vi "BISS_ReadConfigFile.vi"() -> ()   [LabVIEW 2019]
uses:
  DUT_Interface/lv_interface/MHM_1SL_interface.lvlib
panel:
  out "pulEnSsi":u32
  in  "pcFilename":string="test.cfg"
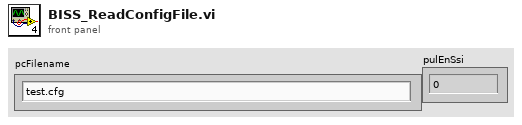
[diagram p1: front panel]
types:
  T1 = enum16{"MHM_NO_INTERFACE", "MHM_MB3U_SPI", "MHM_MB3U_BISS", "MHM_MB4U", "MHM_MB5U"}
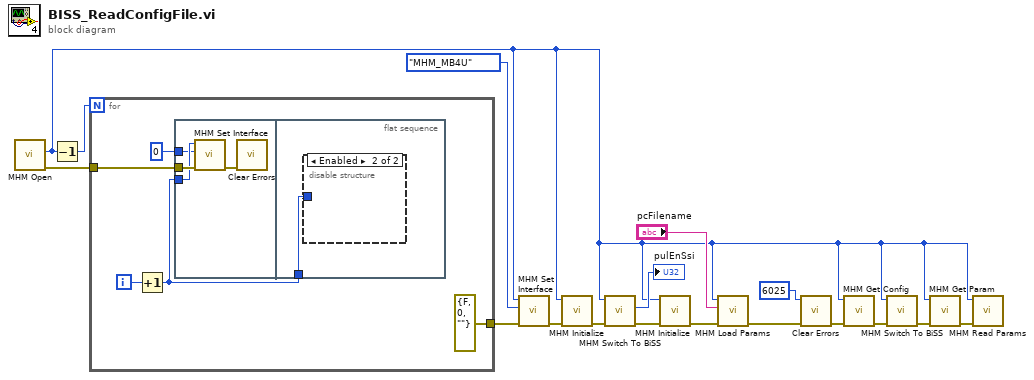
[diagram p0: block diagram]
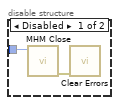
[diagram p2: hidden frame]
diagram:
  n1 = call "MHM Open.vi"() -> ("error out"=w15:errorcluster, "pulMHMHandle"=w4:u32)  [unwired: 9 in, 1 out]
  n2 = Decrement(x=w4) -> (x-1=w10:u32)
  n3 = for {
    N: w10 -> [_]
    tunnel: w15 -> [w21]
    tunnel: [errorcluster {"status"=FALSE, "code"=0, "source"=""} ("error out")] -> w1
    i -> [w20]
    n4 = Increment(x=w20) -> (x+1=w18:i32)
    n5 = flat-sequence {
      tunnel: w21 -> [w26]
      tunnel: w18 -> [w25]
      tunnel: u32 0 ("ulInterface") -> [w24]
      tunnel: w18 -> [w27]
      frame #0 {
        n6 = call "MHM Set Interface.vi"("error in (no error)"=w26, "ulInterface"=w24, "ulMHMHandle"=w25) -> ("error out"=w23:errorcluster)  [unwired: 7 in, 1 out]
        n7 = call <vilib>:"Clear Errors.vi"("error in (no error)"=w23) -> ()  [unwired: 5 in, 2 out]
      }
      frame #1 {
        n8 = disable-structure shown="Enabled" {
          disable-tunnel: w27 -> [w29 _]
          frame Disabled {
            n9 = call "MHM Close.vi"("ulMHMHandle"=w29) -> ("error out"=w28:errorcluster)  [unwired: 9 in, 1 out]
            n10 = call <vilib>:"Clear Errors.vi"("error in (no error)"=w28) -> ()  [unwired: 5 in, 2 out]
          }
          frame Enabled {
          }
        }
      }
    }
  }
  n11 = call "MHM Set Interface.vi"("error in (no error)"=w1, "ulInterface"=T1."MHM_MB4U" ("MHM_InterfaceEnum"), "ulMHMHandle"=w4) -> ("error out"=w5:errorcluster)  [unwired: 7 in, 1 out]
  n12 = call "MHM Initialize.vi"("error in (no error)"=w5, "ulMHMHandle"=w4) -> ("error out"=w3:errorcluster)  [unwired: 8 in, 1 out]
  n13 = call "MHM Switch To BiSS.vi"("error in (no error)"=w3, "ulMHMHandle"=w4) -> ("error out"=w2:errorcluster, "pulEnSsi"=→"pulEnSsi":u32)  [unwired: 7 in, 1 out]
  n14 = call "MHM Initialize.vi"("error in (no error)"=w2, "ulMHMHandle"=w4) -> ("error out"=w16:errorcluster)  [unwired: 8 in, 1 out]
  n15 = call "MHM Load Params.vi"("error in (no error)"=w16, "pcFilename"="pcFilename", "ulMHMHandle"=w4) -> ("error out"=w9:errorcluster)  [unwired: 7 in, 1 out]
  n16 = call <vilib>:"Clear Errors.vi"("error in (no error)"=w9, "specific error code to clear (0: all)"=6025) -> ("error out"=w8:errorcluster)  [unwired: 4 in, 1 out]
  n17 = call "MHM Get Config.vi"("error in (no error)"=w8, "ulMHMHandle"=w4) -> ("error out"=w12:errorcluster)  [unwired: 7 in, 2 out]
  n18 = call "MHM Switch To BiSS.vi"("error in (no error)"=w12, "ulMHMHandle"=w4) -> ("error out"=w13:errorcluster)  [unwired: 7 in, 2 out]
  n19 = call "MHM Get Param.vi"("error in (no error)"=w13, "ulMHMHandle"=w4) -> ("error out"=w14:errorcluster)  [unwired: 7 in, 2 out]
  n20 = call "MHM Read Params.vi"("error in (no error)"=w14, "ulMHMHandle"=w4) -> ()  [unwired: 8 in, 2 out]
